vi "Simulated Acquisition Template (Simulated FPGA VI).vi"() -> ()   [LabVIEW 2016]
uses:
  <vilib>/FPGA/interface/niFpgaViExecutionMode.ctl
  <vilib>/rvi/interface/RandomDataEmulation/nirviRandomDataOpen.vi
  <vilib>/rvi/interface/common/niFpgaCacheSessionInfoDynamic.vi
  <vilib>/rvi/interface/common/dynamic/niFpgaDynamicGetExecutionMode.vi
  <vilib>/FPGAPlugInAG/Dynamic/niLvFpga_Run_Dynamic.vi
  <vilib>/rvi/interface/common/niFpgaWaitOnOcc.vi
  <vilib>/vision/EDVR.llb/IMAQ ImageToEDVR 2D U32.vi
  <vilib>/vision/EDVR.llb/IMAQ ImageToEDVR 2D U8.vi
  <vilib>/rvi/errors/niLvFpgaAdjustHostInterfaceError.vi
  <vilib>/FPGAPlugInAG/Dynamic/niLvFpga_Close_Dynamic.vi
  <vilib>/rvi/interface/nirviOpenFPGA/nirviOpenFPGA.xnode
  TEST TRANSFER.vi
  <vilib>/rvi/interface/nirviMethod/nirviMethod.xnode
  <vilib>/rvi/interface/nirviCloseFPGA/nirviCloseFPGA.xnode
  <vilib>/FPGAPlugInAG/Dynamic/niLvFpga_ConfigureFifo_Dynamic.vi
  <vilib>/rvi/errors/niLvFpgaMergeErrorWithErrorCode.vi
  <vilib>/FPGAPlugInAG/Dynamic/niLvFpga_StartFifo_Dynamic.vi
  <vilib>/FPGAPlugInAG/Dynamic/niLvFpga_WriteFifo_Dynamic.vi
  <vilib>/FPGAPlugInAG/Dynamic/niLvFpga_ReadFifo_Dynamic.vi
panel:
  out "Boolean":bool
  out "output array":u8[][](array[numeric])
  out "Processed Image Count":i32
  in  "Image Folder":path=path "C:/Users/WangPeng/Desktop/for roboRIO/test"
  out "Error Out":errorcluster
  out "Image":T1(plugin-control)
  in  "Stop":bool
  # "Overview: Demonstrates how to cycle through a folder of images and simulate the processing of the image on the FPGA.  This VI is only intended to be used when the FPGA Target is configured to be in the \"Simulation (Simulated I/O)\" Execution Mode.  Simulation is only supported in the \"My Computer\" execution context (i.e. not on a Real-Time target).\nRequirements:\n- LabVIEW FPGA\n- Vision Acquisition Software\n- Vision Development Module\nInstructions:\n1. Select the folder containing the images to use.\n2. Run the VI."
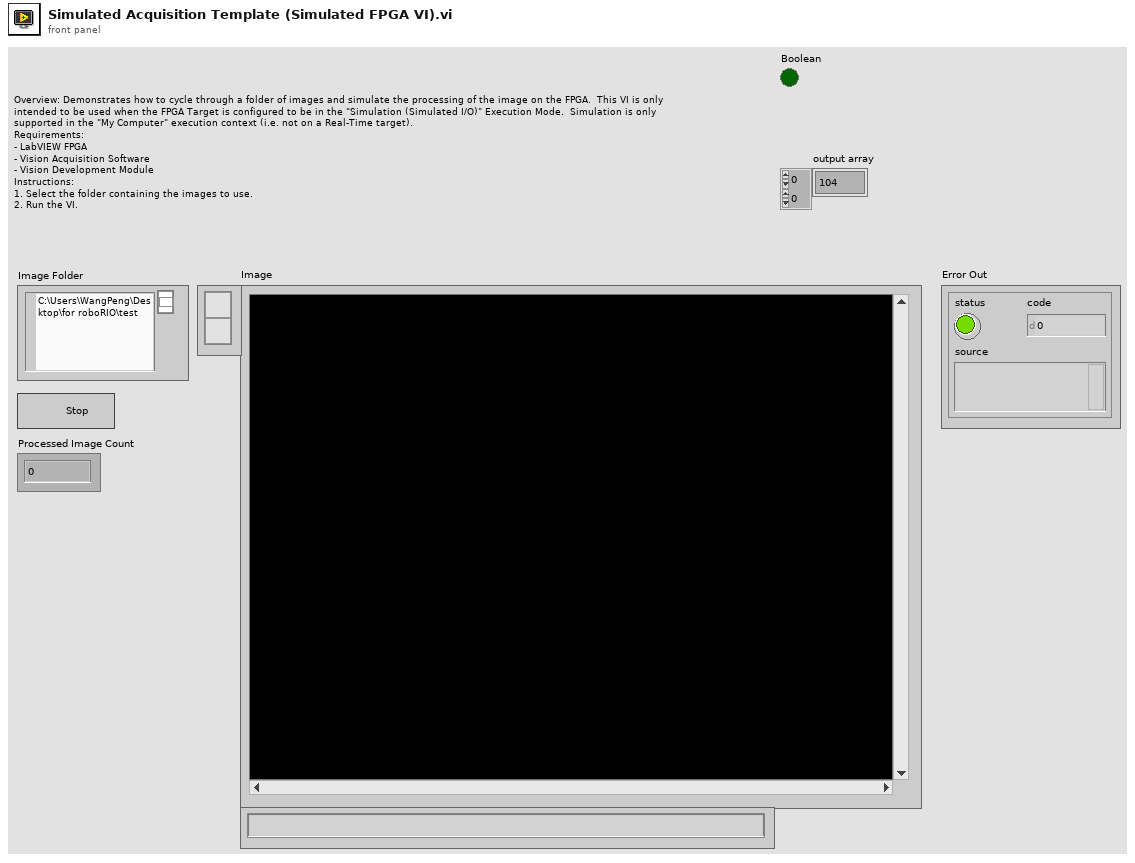
[diagram p1: front panel]
types:
  T1 = typedef "IMAQ Image.ctl" = refnum<image>
  T2 = typedef "niFpgaViExecutionMode.ctl" = enum16{"FPGA Target", "Simulation (Simulated I/O)", "Simulation (Real I/O)", "Third-Party Simulation"}
  T3 = typedef "Image Type" = u32
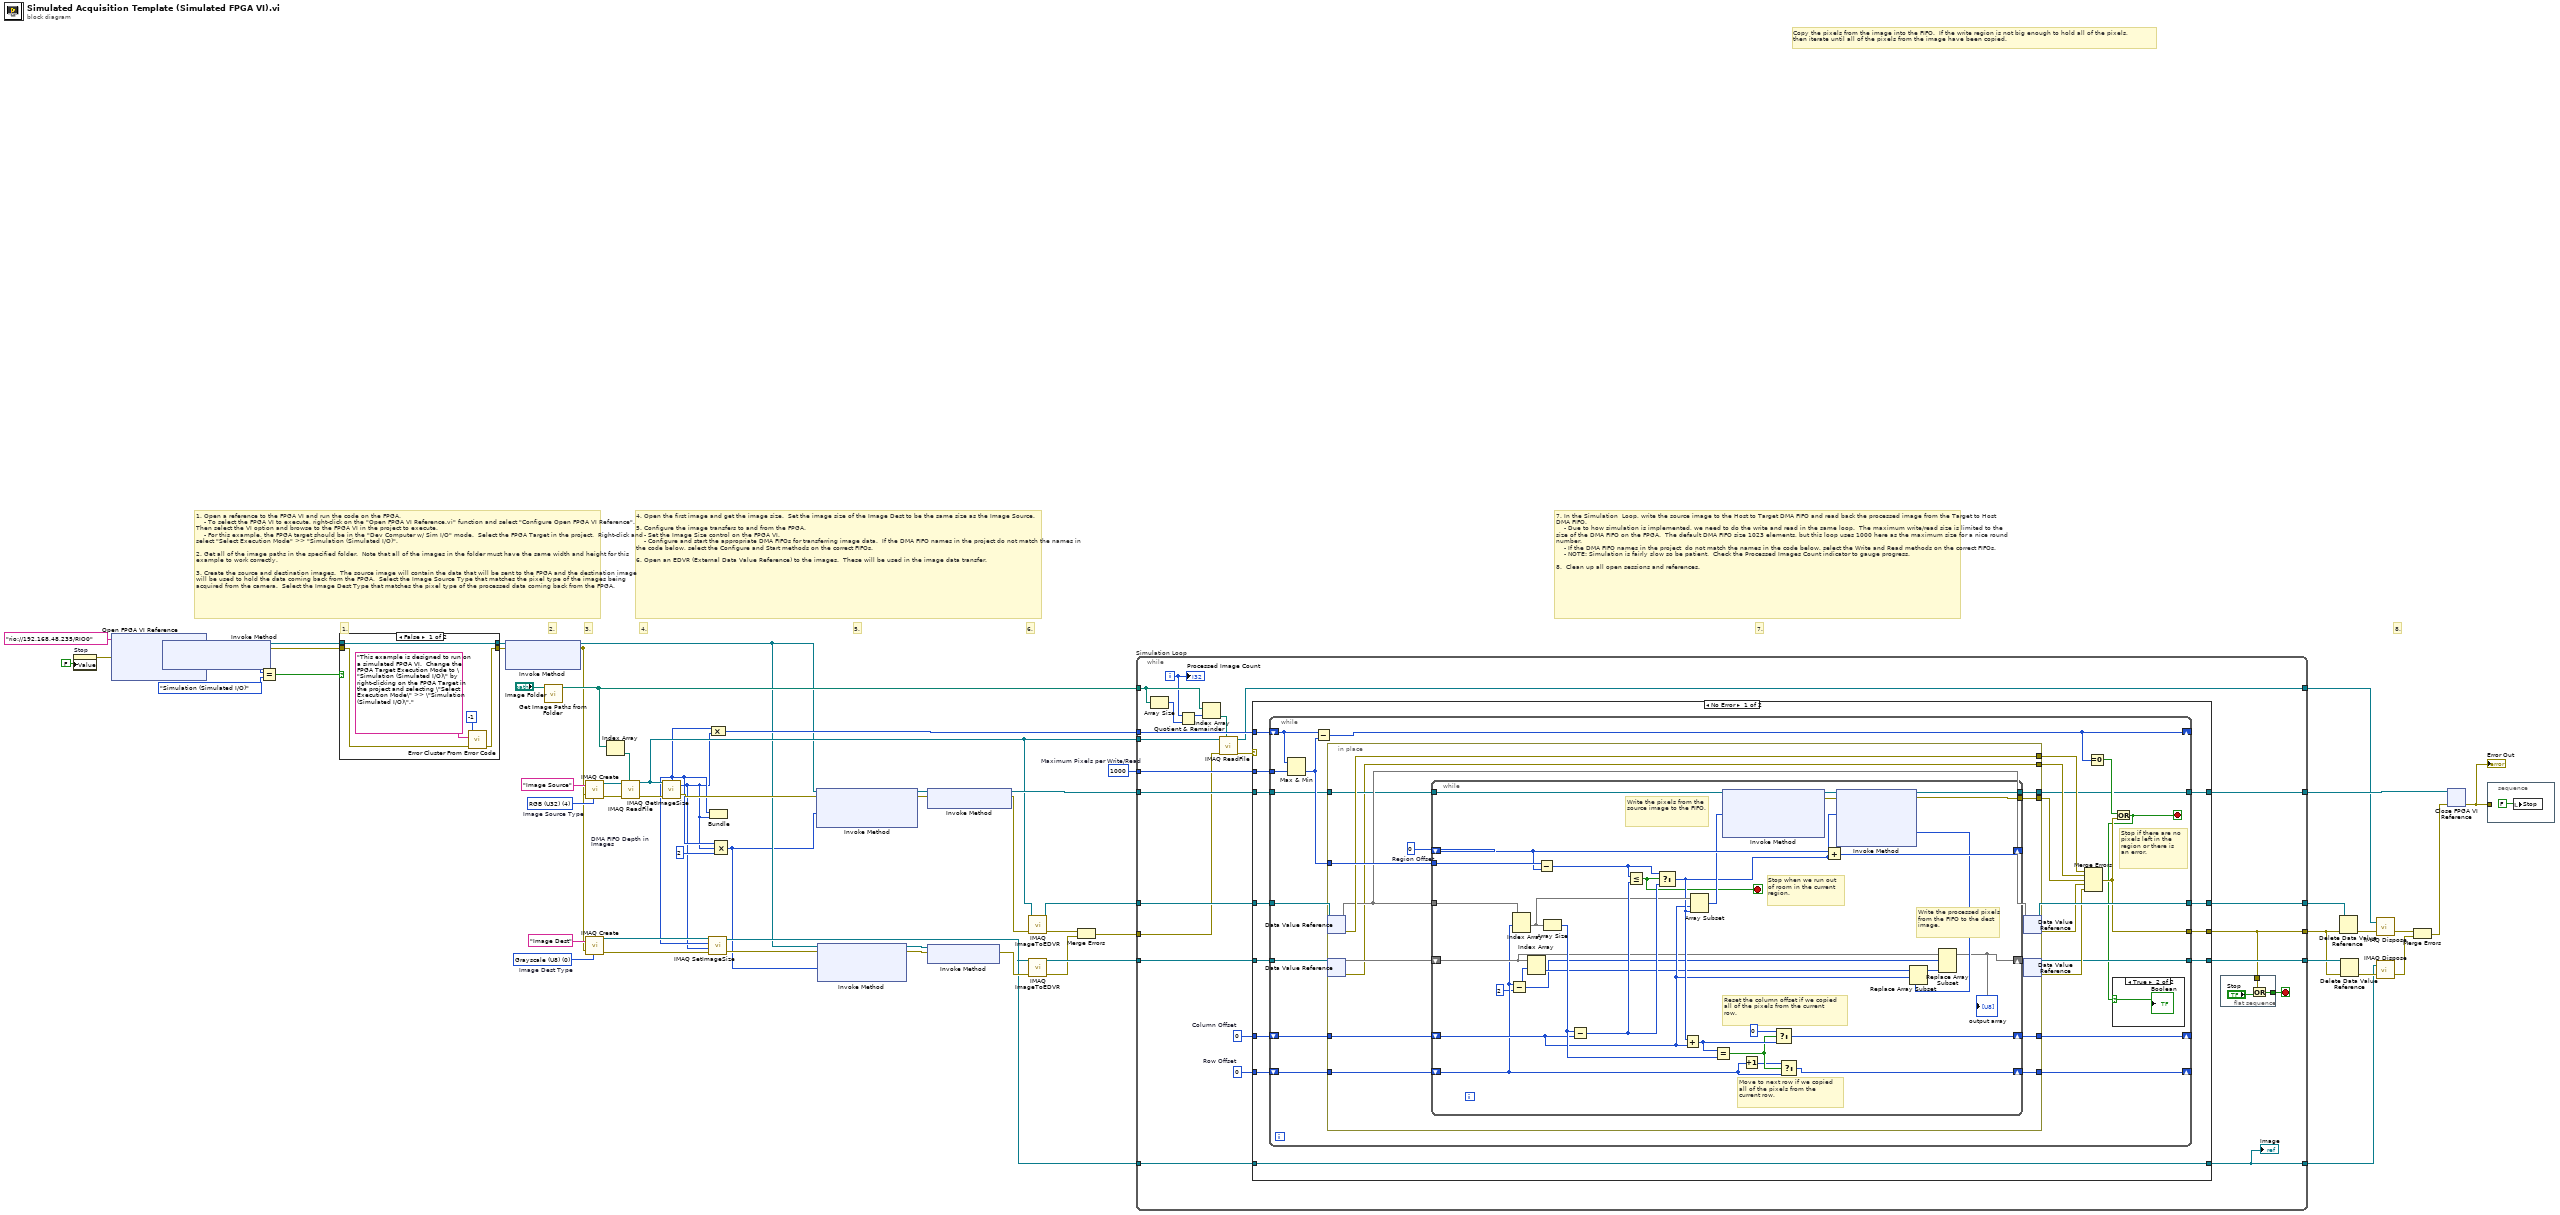
[diagram p0: block diagram]
diagram:
  w24 = u32 1000  # Maximum Pixels per Write/Read
  w48 = u32 2  # DMA FIFO Depth in Images
  w52 = T3 0 items=["Grayscale (U8)", "Grayscale (I16)", "Grayscale (SGL)", "Complex (CSG)", "RGB (U32)", "HSL (U32)", "RGB (U64)", "Grayscale (U16)"]  # Image Dest Type
  w53 = T3 4 items=["Grayscale (U8)", "Grayscale (I16)", "Grayscale (SGL)", "Complex (CSG)", "RGB (U32)", "HSL (U32)", "RGB (U64)", "Grayscale (U16)"]  # Image Source Type
  # "7. In the Simulation  Loop, write the source image to the Host to Target DMA FIFO and read back the processed image from the Target to Host DMA FIFO.  \n    - Due to how simulation is implemented, we need to do the write and read in the same loop.  The maximum write/read size is limited to the size of the DMA FIFO on the FPGA.  The default DMA FIFO size 1023 elements, but this loop uses 1000 here as the maximum size for a nice round number.\n    - If the DMA FIFO names in the project  do not match the names in the code below, select the Write and Read methods on the correct FIFOs. \n    - NOTE: Simulation is fairly slow so be patient.  Check the Processed Images Count indicator to gauge progress.\n\n8.  Clean up all open sessions and references."
  # "4. Open the first image and get the image size.  Set the image size of the Image Dest to be the same size as the Image Source.\n\n5. Configure the image transfers to and from the FPGA.  \n    - Set the Image Size control on the FPGA VI. \n    - Configure and start the appropriate DMA FIFOs for transferring image data.  If the DMA FIFO names in the project do not match the names in the code below, select the Configure and Start methods on the correct FIFOs.\n\n6. Open an EDVR (External Data Value Reference) to the images.  These will be used in the image data transfer."
  # "Copy the pixels from the image into the FIFO.  If the write region is not big enough to hold all of the pixels,\nthen iterate until all of the pixels from the image have been copied."
  # "1. Open a reference to the FPGA VI and run the code on the FPGA.\n    - To select the FPGA VI to execute, right-click on the \"Open FPGA VI Reference.vi\" function and select \"Configure Open FPGA VI Reference\".  Then select the VI option and browse to the FPGA VI in the project to execute.\n    - For this example, the FPGA target should be in the \"Dev Computer w/ Sim I/O\" mode.  Select the FPGA Target in the project.  Right-click and select \"Select Execution Mode\" >> \"Simulation (Simulated I/O)\".\n\n2. Get all of the image paths in the specified folder.  Note that all of the images in the folder must have the same width and height for this example to work correctly.\n\n3. Create the source and destination images.  The source image will contain the data that will be sent to the FPGA and the destination image will be used to hold the data coming back from the FPGA.  Select the Image Source Type that matches the pixel type of the images being acquired from the camera.  Select the Image Dest Type that matches the pixel type of the processed data coming back from the FPGA."
  # "8."
  # "7."
  # "6."
  # "5."
  # "4."
  # "3."
  # "2."
  # "1."
  n1 = property on="Stop" class="Bool (strict)"("Value"=FALSE ("Stop")) -> (error out=w57:errorcluster)  [unwired: 2 in, 1 out]
  n2 = xnode "Open FPGA VI Reference"("error in"=w57, "resource name"=tag "rio://192.168.48.235/RIO0") -> ("FPGA VI Reference Out"=w7:refnum<k20>, "error out"=w6:errorcluster)
  n3 = xnode "Invoke Method"("FPGA VI Reference In"=w7, "error in"=w6) -> ("FPGA VI Reference Out"=w10:refnum<k20>, "error out"=w9:errorcluster, "FPGA VI Execution Mode"=w14:T2)
  n4 = Equal?(x=w14, y=niFpgaViExecutionMode."Simulation (Simulated I/O)" ("FPGA VI Execution Mode")) -> (x = y?=w12:bool)
  n5 = case shown="False" w12 {
    tunnel: [w65 w67] -> w11
    tunnel: w10 -> [w65 w67]
    tunnel: w9 -> [w61 w66]
    tunnel: [w64 w66] -> w8
    frame False {
      n6 = call <vilib>:"Error Cluster From Error Code.vi"("error in (no error)"=w61, "error message (\"\")"="This example is designed to run on a simulated FPGA VI.  Change the FPGA Target Execution Mode to \"Simulation (Simulated I/O)\" by right-clicking on the FPGA Target in the project and selecting \"Select Execution Mode\" >> \"Simulation (Simulated I/O)\"." ("error message (\"\")"), "error code (0)"=-1) -> ("error out"=w64:errorcluster)  [unwired: 6 in]
    }
    frame True {
    }
  }
  n7 = xnode "Invoke Method"("FPGA VI Reference In"=w11, "error in"=w8) -> ("FPGA VI Reference Out"=w2:refnum<k20>, "error out"=w5:errorcluster)  [unwired: 1 in]
  n8 = call "Get Image Paths from Folder.vi"("Image Folder"="Image Folder") -> ("Image Paths"=w17:path[])  [unwired: 10 in]
  n9 = call "IMAQ Create"("Image Name"="Image Source", "Image Type"=w53, "error in (no error)"=w5) -> ("New Image"=w22:T1, "error out"=w21:errorcluster)  [unwired: 2 in]
  n10 = call "IMAQ Create"("Image Name"="Image Dest", "Image Type"=w52, "error in (no error)"=w5) -> ("New Image"=w51:T1, "error out"=w50:errorcluster)  [unwired: 2 in]
  n11 = Index Array(array=w17) -> (element=w18:path)  [unwired: 1 in]
  n12 = call "IMAQ ReadFile"("File Path"=w18, "error in (no error)"=w21, "Image"=w22) -> ("error out"=w19:errorcluster, "Image Out"=w20:T1)  [unwired: 4 in, 3 out]
  n13 = call "IMAQ GetImageSize"("Image"=w20, "error in (no error)"=w19) -> ("Y Resolution"=w3:i32, "X Resolution"=w4:i32, "error out"=w49:errorcluster)  [unwired: 2 in]
  n14 = call "IMAQ SetImageSize"("error in (no error)"=w50, "Y Resolution"=w3, "X Resolution"=w4, "Image"=w51) -> ("error out"=w43:errorcluster, "Image Out"=w27:T1)  [unwired: 1 in]
  n15 = Bundle("X Resolution"=w4, "Y Resolution"=w3) -> ()  [unwired: 1 in, 1 out]
  n16 = Compound Arithmetic op=MULTIPLY(w4, w3) -> (w28:i32)
  n17 = Compound Arithmetic op=MULTIPLY(w4, w3, w48) -> (w1:u32)
  n18 = xnode "Invoke Method"("FPGA VI Reference In"=w2, "error in"=w49, "Requested Depth"=w1) -> ("FPGA VI Reference Out"=w47:refnum<k20>, "error out"=w46:errorcluster)  [unwired: 1 out]
  n19 = xnode "Invoke Method"("FPGA VI Reference In"=w2, "error in"=w43, "Requested Depth"=w1) -> ("FPGA VI Reference Out"=w45:refnum<k20>, "error out"=w44:errorcluster)  [unwired: 1 out]
  n20 = xnode "Invoke Method"("FPGA VI Reference In"=w47, "error in"=w46) -> ("FPGA VI Reference Out"=w29:refnum<k20>, "error out"=w41:errorcluster)
  n21 = xnode "Invoke Method"("FPGA VI Reference In"=w45, "error in"=w44) -> ("error out"=w39:errorcluster)  [unwired: 1 out]
  n22 = call-poly <vilib>:"IMAQ ImageToEDVR.vi"("error out"=w41, "Image"=w20) -> ("error out"=w40:errorcluster, "EDVR 2D U32"=w42:refnum<data-value>)  [unwired: 7 in, 1 out]
  n23 = call-poly <vilib>:"IMAQ ImageToEDVR.vi"("error in (no error)"=w39, "Image"=w27) -> ("error out"=w37:errorcluster, "EDVR 2D U8"=w38:refnum<data-value>)  [unwired: 7 in, 1 out]
  n24 = Merge Errors(w40, w37) -> (w16:errorcluster)
  n25 = while "Simulation Loop" {
    tunnel: [w80] -> w33
    tunnel: w20 -> [w70]
    tunnel: w29 -> [w87]
    tunnel: [w68] -> w15
    tunnel: w42 -> [w88]
    tunnel: w38 -> [w89]
    tunnel: w27 -> [w83]
    tunnel: [w81] -> w36
    tunnel: [w82] -> w34
    tunnel: w28 -> [w86]
    tunnel: [w79] -> w26
    tunnel: [w78] -> w25
    tunnel: w24 -> [w77]
    tunnel: w17 -> [w73]
    tunnel: w16 -> [w72]
    i -> [w69]
    stop <- w90 stop-if-true
    w84 = u32 0  # Row Offset
    w85 = u32 0  # Column Offset
    n26 = Array Size(array=w73) -> (size(s)=w76:i32)
    n27 = Quotient & Remainder(x=w69, y=w76) -> (x-y*floor(x/y)=w74:i32)  [unwired: 1 out]
    n28 = Index Array(array=w73, index=w74) -> (element=w75:path)
    n29 = call "IMAQ ReadFile"("File Path"=w75, "error in (no error)"=w72, "Image"=w70) -> ("error out"=w71:errorcluster, "Image Out"=w68:T1)  [unwired: 4 in, 3 out]
    n30 = case shown="No Error" w71 {
      selector: w71 -> [_ w175]
      tunnel: w86 -> [w102 _]
      tunnel: w88 -> [w101 w174]
      tunnel: w85 -> [w100 _]
      tunnel: w84 -> [w99 _]
      tunnel: w87 -> [w98 w171]
      tunnel: [w97 w175] -> w80
      tunnel: [w96 w174] -> w81
      tunnel: w77 -> [w95 _]
      tunnel: w89 -> [w94 w172]
      tunnel: w83 -> [w93 w173]
      tunnel: [w93 w173] -> w79
      tunnel: [w92 w172] -> w82
      tunnel: [w91 w171] -> w78
      frame No Error {
        n31 = while {
          shift-right: [w118] -> _
          shift-left: w102 -> [w115]
          tunnel: w101 -> [w124]
          shift-right: [w120] -> _
          shift-left: w100 -> [w122]
          shift-right: [w123] -> _
          shift-left: w99 -> [w121]
          tunnel: w98 -> [w112]
          tunnel: [w119] -> w96
          tunnel: [w117] -> w97
          tunnel: w95 -> [w114]
          tunnel: w94 -> [w111]
          tunnel: [w105] -> w92
          tunnel: [w104] -> w91
          stop <- w103 stop-if-true
          # "Stop if there are no\npixels left in the \nregion or there is\nan error."
          n32 = Max & Min(x=w115, y=w114) -> (min(x,y)=w113:u32)  [unwired: 1 out]
          n33 = Subtract(x=w115, y=w113) -> (x-y=w118:u32)
          n34 = in-place {
            in-place-border: w113 -> [w137]
            in-place-border: [w139] -> w123
            in-place-border: w122 -> [w136]
            in-place-border: w121 -> [w133]
            in-place-border: [w135] -> w120
            in-place-border: [w134] -> w108
            in-place-border: w112 -> [w131]
            in-place-border: [w128] -> w107
            in-place-border: [w127] -> w106
            in-place-border: [w126] -> w104
            w138 = u32 0  # Region Offset
            n35 = in-place-dvr #1(w124) -> (w132:u32[][], w134:errorcluster)
            n36 = in-place-dvr #2(w111) -> (w130:u8[][], w128:errorcluster)
            n37 = while {
              tunnel: w132 -> [w158]
              shift-right: [w168] -> _
              shift-left: w138 -> [w167]
              tunnel: w137 -> [w170]
              shift-right: [w162] -> w135
              shift-left: w136 -> [w151]
              shift-right: [w159] -> w139
              shift-left: w133 -> [w144]
              tunnel: w131 -> [w142]
              shift-right: [w147] -> w129
              shift-left: w130 -> [w148]
              tunnel: [w146] -> w127
              tunnel: [w145] -> w126
              stop <- w140 stop-if-true
              # "Write the processed pixels from the FIFO to the dest image."
              # "Stop when we run out\nof room in the current\nregion."
              # "Write the pixels from the source image to the FIFO."
              # "Reset the column offset if we copied\nall of the pixels from the current\nrow."
              # "Move to next row if we copied\nall of the pixels from the\ncurrent row."
              n38 = Subtract(x=w144, y=u32 2) -> (x-y=w143:u32)
              n39 = Index Array(array=w158, index (row)=w144) -> (element=w157:u32[])  [unwired: 1 in]
              n40 = Index Array(array=w148, index (row)=w143) -> (element=w149:u8[])  [unwired: 1 in]
              n41 = Subtract(x=w170, y=w167) -> (x-y=w169:u32)
              n42 = Array Size(array=w157) -> (size(s)=w166:i32)
              n43 = Subtract(x=w166, y=w151) -> (x-y=w165:u32)
              n44 = Less Or Equal?(x=w169, y=w165) -> (x <= y?=w140:bool)
              n45 = Select(t=w169, s=w140, f=w165) -> (s? t:f=w153:u32)
              n46 = Add(x=w153, y=w151) -> (x+y=w163:u32)
              n47 = Array Subset(array=w157, index=w151, length=w153) -> (w156:u32[])
              n48 = Equal?(x=w163, y=w166) -> (x = y?=w161:bool)
              n49 = xnode "Invoke Method"("FPGA VI Reference In"=w142, "Data"=w156) -> ("FPGA VI Reference Out"=w155:refnum<k20>, "error out"=w154:errorcluster)  [unwired: 2 in, 1 out]
              n50 = Increment(x=w144) -> (x+1=w160:u32)
              n51 = Select(t=u32 0 ("Elements In Region"), s=w161, f=w163) -> (s? t:f=w162:u32)
              n52 = Select(t=w160, s=w161, f=w144) -> (s? t:f=w159:u32)
              n53 = Add(x=w167, y=w153) -> (x+y=w168:u32)
              n54 = xnode "Invoke Method"("FPGA VI Reference In"=w155, "error in"=w154, "Number of Elements"=w153) -> ("FPGA VI Reference Out"=w145:refnum<k20>, "error out"=w146:errorcluster, "Data"=w150:u8[])  [unwired: 1 in, 1 out]
              n55 = Replace Array Subset(array=w149, new element=w150, index=w151) -> (w152:u8[])
              n56 = Replace Array Subset(array=w148, new element=w152, index (row)=w143) -> (w147:u8[][])  [unwired: 1 in]
              "output array" <- w147
            }
            n57 = in-place-dvr #1(w132) -> (w119:refnum<data-value>, w110:errorcluster)
            n58 = in-place-dvr #2(w129) -> (w105:refnum<data-value>, w109:errorcluster)
          }
          n59 = Merge Errors(w108, w107, w106, w110, w109) -> (w117:errorcluster)
          n60 = Equal To 0?(x=w118) -> (x = 0?=w116:bool)
          n61 = Or(x=w116, y=w117) -> (x .or. y?=w103:bool)
          n62 = case shown="True" w103 {
            selector: w103 -> [_ w125]
            frame False {
            }
            frame True {
              "Boolean" <- w125
            }
          }
        }
      }
      frame Error {
      }
    }
    "Image" <- w79
    n63 = flat-sequence {
      tunnel: [w177] -> w90
      tunnel: w80 -> [w176]
      frame #0 {
        n64 = Or(x=w176, y="Stop") -> (x .or. y?=w177:bool)
      }
    }
    "Processed Image Count" <- w69
  }
  n65 = Delete Data Value Reference(data value reference=w36, error in=w33) -> (error out=w35:errorcluster)  [unwired: 1 out]
  n66 = Delete Data Value Reference(data value reference=w34, error in=w33) -> (error out=w32:errorcluster)  [unwired: 1 out]
  n67 = call "IMAQ Dispose"("Image"=w15, "error in (no error)"=w35) -> ("error out"=w30:errorcluster)  [unwired: 4 in]
  n68 = call "IMAQ Dispose"("Image"=w26, "error in (no error)"=w32) -> ("error out"=w31:errorcluster)  [unwired: 4 in]
  n69 = Merge Errors(w30, w31) -> (w55:errorcluster)
  n70 = xnode "Close FPGA VI Reference"("FPGA VI Reference In"=w25, "error in"=w55) -> ("error out"=w54:errorcluster)
  "Error Out" <- w54
  n71 = stacked-sequence {
    tunnel: w54 -> [_]
    frame #0 {
      n72 = local write "Stop"(FALSE ("Stop")) -> ()
    }
  }
